vi "SMO.InstrumentDriver.TestLauncher.vi"() -> ()   [LabVIEW 2013, in "SMO.InstrumentDriver.lvclass"]
doc: "JKI State Machine Objects (SMO) 1.0.0.5\nJKI - JKI\nCopyright (c) 2016, JKI"
uses:
  SMO.InstrumentDriver.lvclass
  Typedefs/WriteData.ctl
  Typedefs/Configuration--Cluster.ctl
  <vilib>/JKI/JKI SMO/SMO/Typedefs/SMOState --Enum.ctl
  <vilib>/JKI/JKI SMO/SMO/SMO.lvclass
panel:
  in  "Write":bool
  in  "Data to Write":T1
  in  "Read Now":bool
  out "Measurement":dbl
  in  "Self Test":bool
  in  "Clear Device":bool
  out "error out":errorcluster
  in  "Stop":bool
  # "Intrument Driver Test Launcher"
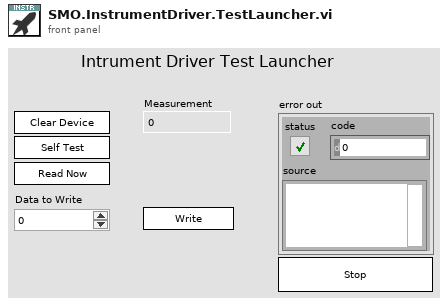
[diagram p1: front panel]
types:
  T1 = typedef "SMO.InstrumentDriver.lvclass/WriteData.ctl" = dbl
  T2 = typedef "SMO.InstrumentDriver.lvclass/Configuration--Cluster.ctl" = cluster{"Polling Rate (ms)":i32}
  T3 = typedef "SMO.lvclass/Public Events.ctl" = cluster{"Error":refnum<user-event>, "State":refnum<user-event>}
  T4 = typedef "SMO.InstrumentDriver.lvclass/PublicEvents--Cluster.ctl" = cluster{"Value Changed":refnum<user-event>}
  T5 = cluster{"Event Registration Refnum":refnum<event-registration>}
  T6 = typedef "SMO.lvclass/SMOState --Enum.ctl" = enum16{"unknown", "Created", "Started", "Stopped"}
  T7 = typedef "SMO.InstrumentDriver.lvclass/ReadData.ctl" = dbl
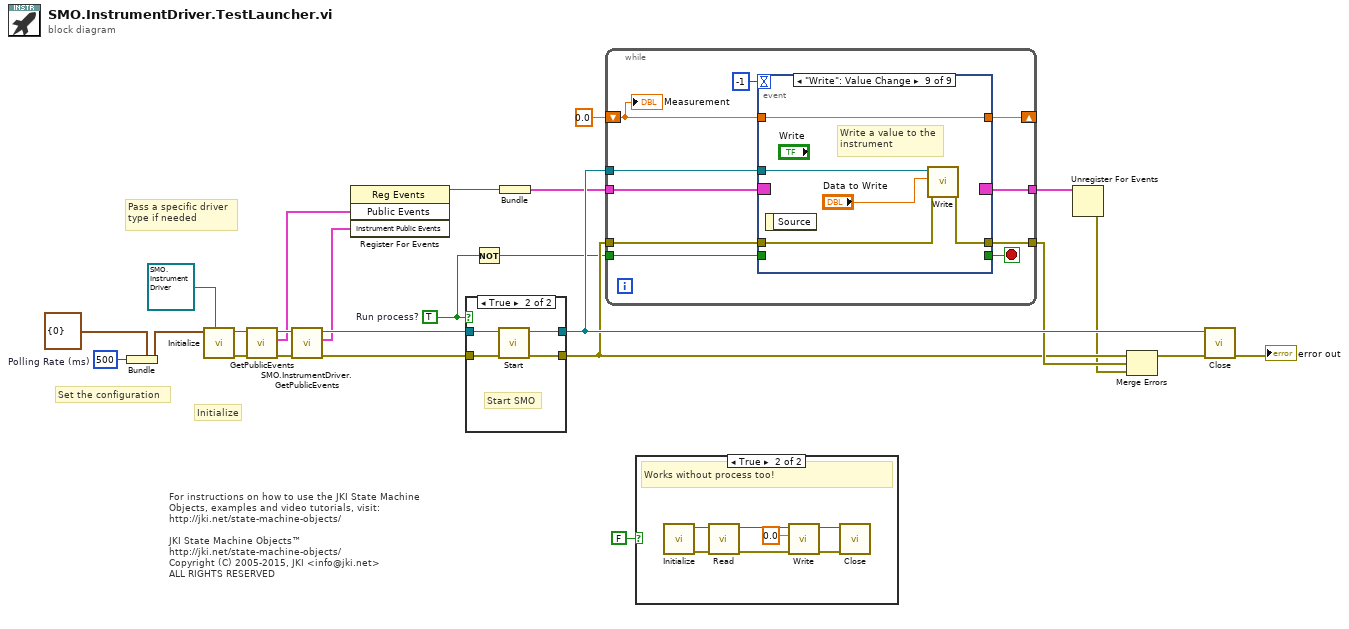
[diagram p0: block diagram]
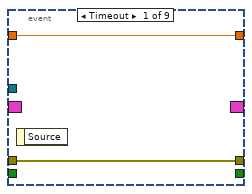
[diagram p4: hidden frame]
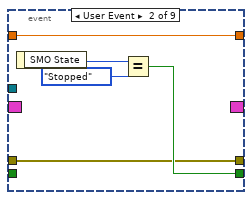
[diagram p5: hidden frame]
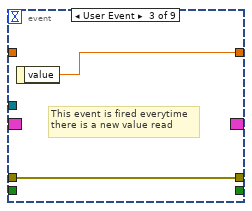
[diagram p6: hidden frame]
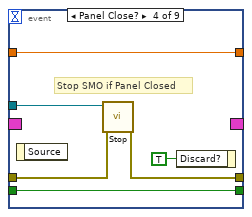
[diagram p7: hidden frame]
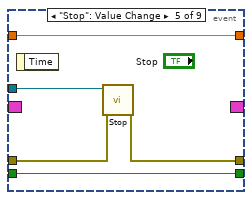
[diagram p8: hidden frame]
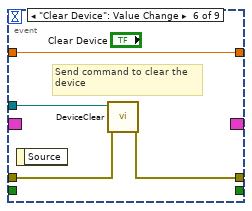
[diagram p9: hidden frame]
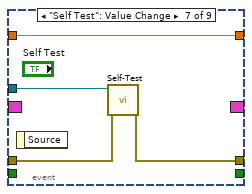
[diagram p10: hidden frame]
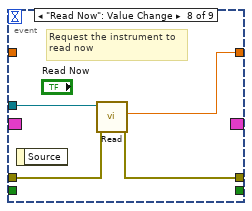
[diagram p11: hidden frame]
diagram:
  w1 = 500  # Polling Rate (ms)
  w6 = TRUE  # Run process?
  # "Set the configuration"
  # "Initialize"
  # "Pass a specific driver\ntype if needed"
  # "For instructions on how to use the JKI State Machine Objects, examples and video tutorials, visit:\nhttp://jki.net/state-machine-objects/\n\nJKI State Machine Objects™\nhttp://jki.net/state-machine-objects/\nCopyright (C) 2005-2015, JKI <info@jki.net>\nALL RIGHTS RESERVED"
  n1 = Bundle(cluster=T2 {"Polling Rate (ms)"=0} ("Configuration"), "Polling Rate (ms)"=w1) -> (w2:T2)
  n2 = call "Initialize.vi"("SMO.InstrumentDriver in"=refnum<class "SMO.InstrumentDriver.lvclass"> refnum, "Configuration"=w2) -> ("error out"=w22:errorcluster, "SMO.InstrumentDriver out"=w21:refnum<class "SMO.InstrumentDriver.lvclass">)  [unwired: 7 in, 1 out]
  n3 = call <vilib>:"GetPublicEvents.vi"("error in (no error)"=w22, "SMO"=w21) -> ("error out"=w15:errorcluster, "Public Events"=w13:T3, "SMO out"=w14:refnum<class "SMO.InstrumentDriver.lvclass">)  [unwired: 7 in]
  n4 = call "SMO.InstrumentDriver.GetPublicEvents.vi"("error in (no error)"=w15, "SMO.Instrument"=w14) -> ("error out"=w19:errorcluster, "Instrument Public Events"=w17:T4, "SMO.Instrument out"=w18:refnum<class "SMO.InstrumentDriver.lvclass">)  [unwired: 7 in]
  n5 = register-events(w13, w17) -> (reference out=w16:refnum<event-registration>)  [unwired: 2 in, 1 out]
  n6 = case shown="True" w6 {
    tunnel: [w27 w31] -> w23
    tunnel: w19 -> [w26 w30]
    tunnel: w18 -> [w27 w29]
    tunnel: [w26 w28] -> w9
    frame False {
    }
    frame True {
      # "Start SMO"
      n7 = call <vilib>:"Start.vi"("error in (no error)"=w30, "SMO"=w29) -> ("error out"=w28:errorcluster, "SMO out"=w31:refnum<class "SMO.InstrumentDriver.lvclass">)  [unwired: 8 in]
    }
  }
  n8 = Not(x=w6) -> (.not. x?=w5:bool)
  n9 = Bundle("Event Registration Refnum"=w16) -> (w11:T5)  [unwired: 1 in]
  n10 = while {
    tunnel: w11 -> [w38]
    tunnel: [w37] -> w12
    tunnel: w23 -> [w36]
    tunnel: w9 -> [w39]
    tunnel: [w40] -> w10
    shift-right: [w34] -> _
    shift-left: 0.0 -> [w32]
    tunnel: w5 -> [w33]
    stop <- w41 stop-if-true
    n11 = event shown="[8] \"Write\": Value Change" {
      selector: w38 -> [_ _ _ _ _ _ _ _ _]
      dyn-events: [_ _ _ _ _ _ _ _ _] -> w37
      timeout: -1 -> [_ _ _ _ _ _ _ _ _]
      tunnel: [_ w46 _ w51 w57 _ _ _ _] -> w41
      tunnel: w36 -> [_ _ _ w56 w61 w65 w69 w73 w78]
      tunnel: [w43 w45 w50 w55 w60 w63 w67 w71 w76] -> w40
      tunnel: w39 -> [w43 w45 w50 w54 w59 w64 w68 w72 w77]
      tunnel: w32 -> [w42 w44 _ w52 w58 w62 w66 _ w75]
      tunnel: [w42 w44 w49 w52 w58 w62 w66 w70 w75] -> w34
      tunnel: w33 -> [_ _ _ w51 w57 _ _ _ _]
      event Timeout {
        n12 = event-data() -> ()  [unwired: 1 in, 1 out]
      }
      event User Event {
        n13 = event-data() -> ("SMO State"=w48:T6)  [unwired: 1 in]
        n14 = Equal?(x=w48, y=SMOState_--Enum."Stopped") -> (x = y?=w46:bool)
      }
      event User Event {
        # "This event is fired everytime\nthere is a new value read"
        n15 = event-data() -> ("value"=w49:T7)  [unwired: 1 in]
      }
      event Panel Close? {
        # "Stop SMO if Panel Closed"
        n16 = event-data() -> ()  [unwired: 1 in, 1 out]
        n17 = call <vilib>:"Stop.vi"("error in (no error)"=w54, "SMO"=w56) -> ("error out"=w55:errorcluster)  [unwired: 8 in, 1 out]
        n18 = event-data("Discard?"=TRUE ("OK")) -> ()  [unwired: 1 in, 1 out]
      }
      event "Stop": Value Change {
        n19 = event-data() -> ()  [unwired: 1 in, 1 out]
        n20 = call <vilib>:"Stop.vi"("error in (no error)"=w59, "SMO"=w61) -> ("error out"=w60:errorcluster)  [unwired: 8 in, 1 out]
      }
      event "Clear Device": Value Change {
        # "Send command to clear the\ndevice"
        n21 = event-data() -> ()  [unwired: 1 in, 1 out]
        n22 = call "DeviceClear.vi"("error in (no error)"=w64, "SMO.Instrument"=w65) -> ("error out"=w63:errorcluster)  [unwired: 8 in, 1 out]
      }
      event "Self Test": Value Change {
        n23 = event-data() -> ()  [unwired: 1 in, 1 out]
        n24 = call "Self-Test.vi"("error in (no error)"=w68, "SMO.Instrument"=w69) -> ("error out"=w67:errorcluster)  [unwired: 8 in, 1 out]
      }
      event "Read Now": Value Change {
        # "Request the instrument to\nread now"
        n25 = event-data() -> ()  [unwired: 1 in, 1 out]
        n26 = call "Read.vi"("error in (no error)"=w72, "SMO.Instrument"=w73) -> ("error out"=w71:errorcluster, "value"=w70:T7)  [unwired: 7 in, 1 out]
      }
      event "Write": Value Change {
        # "Write a value to the\ninstrument"
        n27 = event-data() -> ()  [unwired: 1 in, 1 out]
        n28 = call "Write.vi"("error in (no error)"=w77, "Write"="Data to Write", "SMO.InstrumentDriver"=w78) -> ("error out"=w76:errorcluster)  [unwired: 7 in, 1 out]
      }
    }
    "Measurement" <- w32
  }
  n29 = case shown="True" FALSE {
    frame False {
    }
    frame True {
      # "Works without process too!"
      n30 = call "Initialize.vi"() -> ("error out"=w84:errorcluster, "SMO.InstrumentDriver out"=w85:refnum<class "SMO.InstrumentDriver.lvclass">)  [unwired: 9 in, 1 out]
      n31 = call "Read.vi"("error in (no error)"=w84, "SMO.Instrument"=w85) -> ("error out"=w81:errorcluster, "SMO.Instrument out"=w83:refnum<class "SMO.InstrumentDriver.lvclass">)  [unwired: 7 in, 1 out]
      n32 = call "Write.vi"("error in (no error)"=w81, "Write"=T1 0.0, "SMO.InstrumentDriver"=w83) -> ("error out"=w80:errorcluster, "SMO.InstrumentDriver out"=w82:refnum<class "SMO.InstrumentDriver.lvclass">)  [unwired: 7 in]
      n33 = call "Close.vi"("error in (no error)"=w80, "SMO.InstrumentDriver in"=w82) -> ()  [unwired: 9 in, 1 out]
    }
  }
  n34 = Unregister For Events(event registration refnum=w12) -> (error out=w7:errorcluster)  [unwired: 1 in]
  n35 = Merge Errors(w9, w10, w7) -> (w24:errorcluster)
  n36 = call "Close.vi"("error in (no error)"=w24, "SMO.InstrumentDriver in"=w23) -> ("error out"=→"error out":errorcluster)  [unwired: 9 in]
